vi "CRYUpdate Steps.vi"(8 "AddStepsTree":refnum<vi>, 9 "Category Name":string="stimulus.txt", 10 "Step flattened":string, 11 "StepFileName":string="Stimulus") -> (3 "StepFileNameOut":string)   [LabVIEW 2013]
uses:
  CRYProject/CRYProject Editor Global.vi
panel:
  out "UpLimit":i32
  out "DownLimit":i32
  in  "Symbol Index":i32
  in  "Down Step Name":string="stimulus.txt"
  in  "Boolean":bool
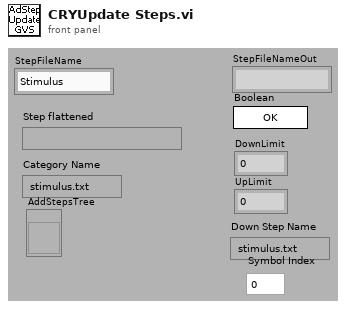
[diagram p1: front panel]
types:
  T1 = cluster{"Content":string, "Name":string, "Level":u32, "Category":string}
  T2 = cluster{"Content":string, "Name":string, "Level":u32, "Category":string}[]
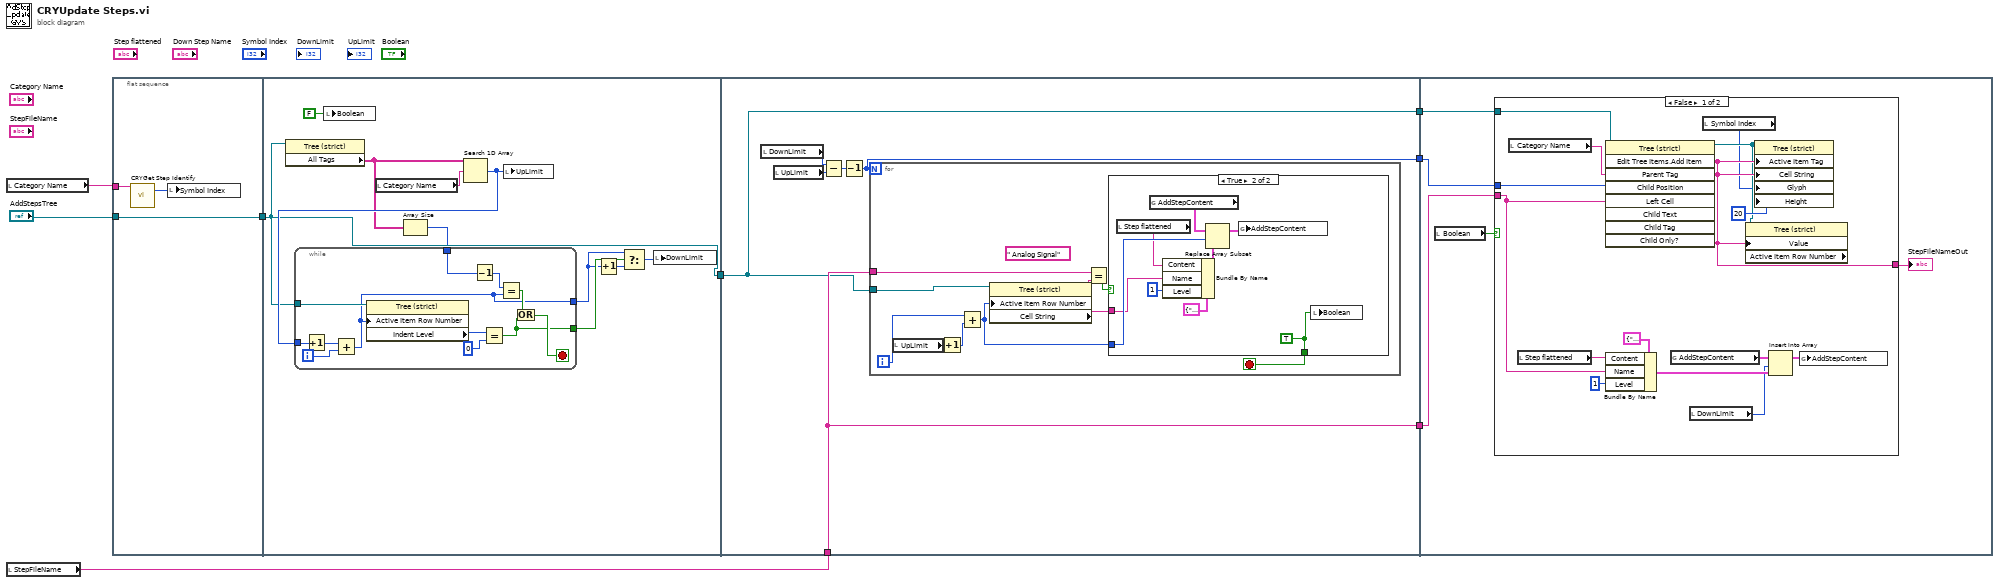
[diagram p0: block diagram]
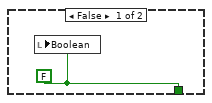
[diagram p2: hidden frame]
diagram:
  n1 = local read "Category Name"() -> (w3:string)
  n2 = local read "StepFileName"() -> (w7:string)
  n3 = flat-sequence {
    tunnel: w3 -> [w10]
    tunnel: [w9] -> w2
    tunnel: "AddStepsTree" -> [w9]
    tunnel: [w18] -> w8
    tunnel: w2 -> [w18]
    tunnel: w8 -> [w35]
    tunnel: w7 -> [w36]
    tunnel: [w34] -> w6
    tunnel: [w36] -> w5
    tunnel: [w35] -> w4
    tunnel: w6 -> [w62]
    tunnel: w5 -> [w61]
    tunnel: w4 -> [w60]
    frame #0 {
      n4 = call "CRYGet Step Identify.vi"("Category Name In"=w10) -> ("Symbol Index"=w11:i32)  [unwired: 3 in, 7 out]
      n5 = local write "Symbol Index"(w11) -> ()
    }
    frame #1 {
      n6 = property class="Tree (strict)"(reference=w18) -> ("All Tags"=w17:string[])  [unwired: 1 in, 2 out]
      n7 = local write "Boolean"(FALSE ("Boolean")) -> ()
      n8 = local read "Category Name"() -> (w20:string)
      n9 = Array Size(array=w17) -> (size(s)=w16:i32)
      n10 = Search 1D Array(1D array=w17, element=w20) -> (index of element=w19:i32)  [unwired: 1 out]
      n11 = while {
        tunnel: w19 -> [w33]
        tunnel: w18 -> [w30]
        tunnel: w16 -> [w24]
        tunnel: [w25] -> w14
        tunnel: [w22] -> w15
        i -> [w32]
        stop <- w26 stop-if-true
        n12 = Increment(x=w33) -> (x+1=w31:i32)
        n13 = Add(x=w31, y=w32) -> (x+y=w25:i32)
        n14 = property class="Tree (strict)"(reference=w30, "Active Item Row Number"=w25) -> ("Indent Level"=w29:i32)  [unwired: 1 in, 2 out]
        n15 = Decrement(x=w24) -> (x-1=w23:i32)
        n16 = Equal?(x=w29, y=0) -> (x = y?=w22:bool)
        n17 = Equal?(x=w23, y=w25) -> (x = y?=w27:bool)
        n18 = Or(x=w27, y=w22) -> (x .or. y?=w26:bool)
      }
      n19 = local write "UpLimit"(w19) -> ()
      n20 = Increment(x=w14) -> (x+1=w13:i32)
      n21 = Select(t=w14, s=w15, f=w13) -> (s? t:f=w12:i32)
      n22 = local write "DownLimit"(w12) -> ()
    }
    frame #2 {
      n23 = local read "DownLimit"() -> (w39:i32)
      n24 = local read "UpLimit"() -> (w38:i32)
      n25 = Subtract(x=w39, y=w38) -> (x-y=w37:i32)
      n26 = Decrement(x=w37) -> (x-1=w34:i32)
      n27 = for {
        N: w34 -> [_]
        tunnel: w36 -> [w43]
        tunnel: w35 -> [w41]
        i -> [w46]
        stop <- w45 stop-if-true
        (unwired) " Analog Signal" ("y")
        n28 = local read "UpLimit"() -> (w48:i32)
        n29 = Increment(x=w48) -> (x+1=w47:i32)
        n30 = Add(x=w46, y=w47) -> (x+y=w42:i32)
        n31 = property class="Tree (strict)"(reference=w41, "Active Item Row Number"=w42) -> ("Cell String"=w40:string)  [unwired: 1 in, 2 out]
        n32 = Equal?(x=w43, y=w40) -> (x = y?=w44:bool)
        n33 = case shown="True" w44 {
          tunnel: [w49 w58] -> w45
          tunnel: w42 -> [_ w55]
          tunnel: w40 -> [_ w53]
          frame False {
            w49 = FALSE
            n34 = local write "Boolean"(w49) -> ()
          }
          frame True {
            w58 = TRUE
            n35 = local read "Step flattened"() -> (w54:string)
            n36 = global read "CRYProject Editor Global.vi" "AddStepContent"() -> (w56:T2)
            n37 = Bundle By Name(cluster=T1 {"Content"="", "Name"="", "Level"=0, "Category"=""}, "Content"=w54, "Name"=w53, "Level"=u32 1) -> (w52:T1)
            n38 = Replace Array Subset(array=w56, new element=w52, index=w55) -> (w57:T2)
            n39 = global write "CRYProject Editor Global.vi" "AddStepContent"(w57) -> ()
            n40 = local write "Boolean"(w58) -> ()
          }
        }
      }
    }
    frame #3 {
      n41 = local read "Boolean"() -> (w63:bool)
      n42 = case shown="False" w63 {
        tunnel: w61 -> [w77 w79]
        tunnel: [w78 w79] -> w59
        tunnel: w62 -> [w66 _]
        tunnel: w60 -> [w76 _]
        frame False {
          n43 = local read "Category Name"() -> (w72:string)
          n44 = local read "Step flattened"() -> (w68:string)
          n45 = invoke on="Invoke Node" class="Tree (strict)" method="Edit Tree Items.Add Item"(reference=w76, "Parent Tag"=w72, "Child Position"=w66, "Left Cell"=w77) -> (reference out=w74:refnum<vi>, "Edit Tree Items:Add Item"=w78:string)  [unwired: 5 in, 7 out]
          n46 = Bundle By Name(cluster=T1 {"Content"="", "Name"="", "Level"=0, "Category"=""}, "Content"=w68, "Name"=w77, "Level"=u32 1) -> (w69:T1)
          n47 = global read "CRYProject Editor Global.vi" "AddStepContent"() -> (w71:T2)
          n48 = local read "DownLimit"() -> (w65:i32)
          n49 = local read "Symbol Index"() -> (w73:i32)
          n50 = property on="Property Node" class="Tree (strict)" props=["Value", "Active Item Row Number"](reference=w74, "Value"=w78) -> ()  [unwired: 1 in, 3 out]
          n51 = property on="Property Node" class="Tree (strict)"(reference=w74, "Active Item Tag"=w78, "Cell String"=w78, "Glyph"=w73, "Height"=20 ("Active Cell:Cell Size:Height")) -> ()  [unwired: 1 in, 2 out]
          n52 = Insert Into Array(array=w71, index=w65, new element=w69) -> (w67:T2)
          n53 = global write "CRYProject Editor Global.vi" "AddStepContent"(w67) -> ()
        }
        frame True {
        }
      }
      "StepFileNameOut" <- w59
    }
  }
